vi "Stop Core.vi"(10 "final error code":i32, 11 "GUI_Dialog_Login in":refnum<class "CalibrationManagerActor.lvclass">) -> (3 "GUI_Dialog_Login out":refnum<class "CalibrationManagerActor.lvclass">)   [LabVIEW 2017, in "CalibrationManagerActor.lvlib" / "CalibrationManagerActor.lvclass"]
doc: "(<B>Filename</B>: Actor Framework.lvlib:Actor.lvclass:Stop Core.vi)\n\nDefines what the actor does before it stops. Use the <B>final error code</B> input to determine whether the actor shut down in response to an error.\n\nBy default, this method does nothing. A descendant class may override it to define behavior, such as shutting down any processes the actor initiated in its override of the Actor Core method."
uses:
  CalibrationManagerActor.lvclass
  CalibrationManagerActor.lvclass/CalibrationManagerActor.ctl
  GUI/GUI/GUI.lvclass
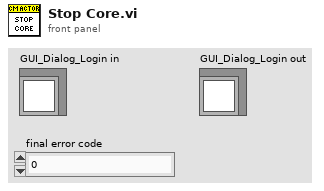
[diagram p1: front panel]
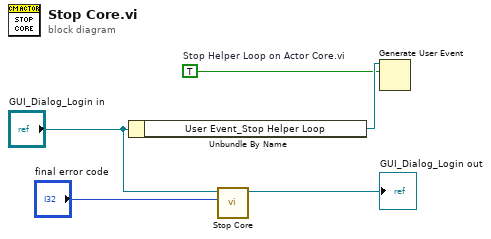
[diagram p0: block diagram]
diagram:
  w1 = TRUE  # Stop Helper Loop on Actor Core.vi
  n1 = Unbundle By Name("GUI_Dialog_Login in") -> ("User Event_Stop Helper Loop"=w2:refnum<user-event>)
  n2 = call-parent "Stop Core.vi"("final error code"="final error code", "Actor in"="GUI_Dialog_Login in") -> ("Actor out"=→"GUI_Dialog_Login out":refnum<class "CalibrationManagerActor.lvclass">)  [unwired: 9 in]
  n3 = Generate User Event(user event=w2, event data cluster=w1) -> ()  [unwired: 2 in, 2 out]
